vi "wfm_feature visable_cursor.vi"(7 "parameter":cluster{"Target":i32, "Coords":T1}, 8 "error in (no error)":errorcluster, 11 "WindowGraph in":refnum<class "wfm_feature.lvclass">) -> (0 "error out":errorcluster, 3 "WindowGraph out":refnum<class "wfm_feature.lvclass">)   [LabVIEW 2018, in "wfm_feature.lvclass"]
uses:
  wfm_feature.lvclass
  <vilib>/Utility/miscctls.llb/LVPoint32TypeDef.ctl
  wfm_feature.lvclass/wfm_feature.ctl
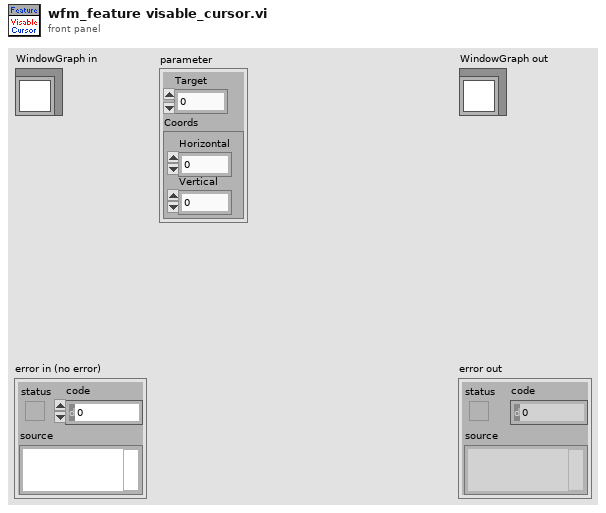
[diagram p1: front panel]
types:
  T1 = typedef "LVPoint32TypeDef.ctl" = cluster{"Horizontal":i32, "Vertical":i32}
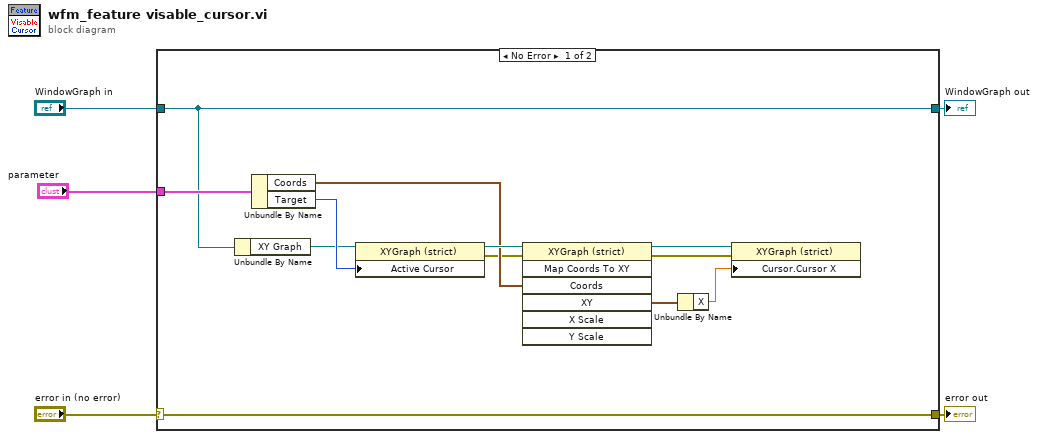
[diagram p0: block diagram]
diagram:
  n1 = case shown="No Error" "error in (no error)" {
    selector: "error in (no error)" -> [w17 w19]
    tunnel: [w17 w19] -> w4
    tunnel: [w7 w18] -> w2
    tunnel: "WindowGraph in" -> [w7 w18]
    tunnel: "parameter" -> [w8 _]
    frame No Error {
      n2 = Unbundle By Name(w7) -> ("XY Graph"=w6:refnum<vi>)
      n3 = Unbundle By Name(w8) -> ("Coords"=w15:T1, "Target"=w14:i32)
      n4 = property class="XYGraph (strict)"(reference=w6, "Active Cursor"=w14) -> (reference out=w16:refnum<vi>, error out=w12:errorcluster)  [unwired: 1 in]
      n5 = invoke class="XYGraph (strict)" method="Map Coords To XY"(reference=w16, error in=w12, "Coords"=w15) -> (reference out=w13:refnum<vi>, error out=w11:errorcluster, "XY"=w10:cluster{"X":dbl, "Y":dbl})  [unwired: 4 in, 4 out]
      n6 = Unbundle By Name(w10) -> ("X"=w9:dbl)
      n7 = property class="XYGraph (strict)"(reference=w13, error in=w11, "Cursor.Cursor X"=w9) -> ()  [unwired: 2 out]
    }
    frame Error {
    }
  }
  "error out" <- w4
  "WindowGraph out" <- w2
